vi "IFF_OneLine.vi"(0 "Ztest":dbl, 1 "Slices":cluster{"HighSlice":T1[], "LowSlice":T1[]}, 2 "TriangleInfo":T4, 5 "Sampling":T3, 7 "X":cluster{"Xmin":dbl, "Xmax":dbl}, 9 "DirVecs":dbl[][](array[numeric]), 11 "Y":dbl, 12 "PixSize(mm)":dbl) -> (4 "LineOut":dbl[](array[numeric]))   [LabVIEW 2014]
uses:
  TypeDefs/Poly2DwSlope.ctl
  TypeDefs/Point2DwSlope.ctl
  <vilib>/Analysis/baseanly.llb/Mean (DBL).vi
  <vilib>/Analysis/NI_AALBase.lvlib
panel:
  out "Waveform Graph":dbl[](graph)
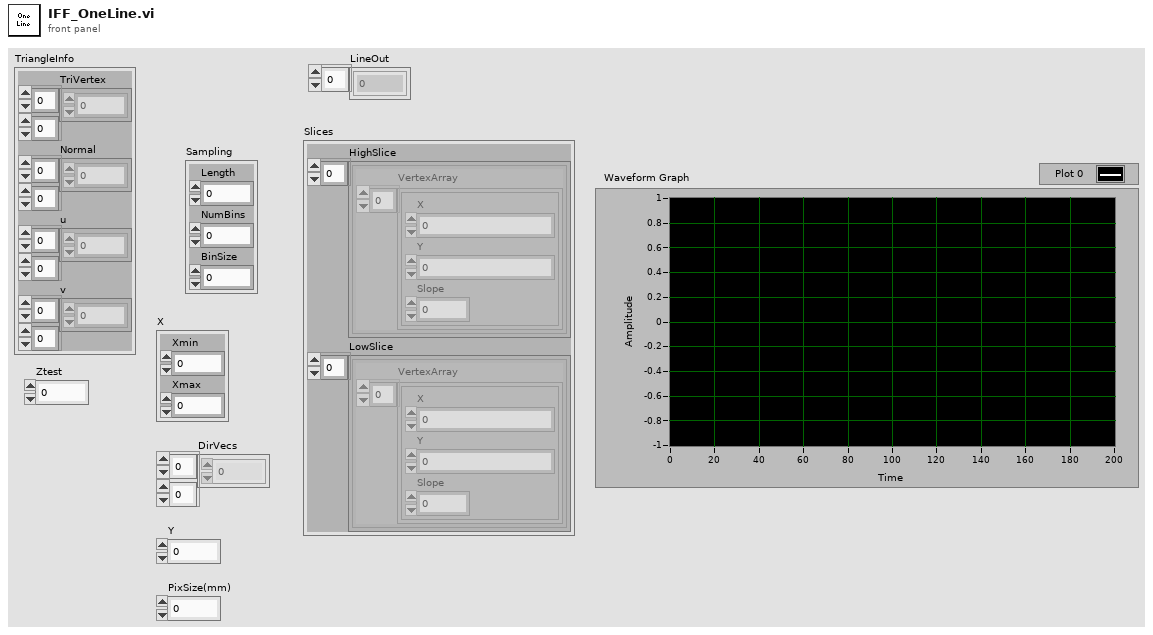
[diagram p1: front panel]
types:
  T1 = typedef "Poly2DwSlope.ctl" = cluster{"VertexArray":T2[]}
  T2 = typedef "Point2DwSlope.ctl" = cluster{"X":sgl, "Y":sgl, "Slope":dbl}
  T3 = cluster{"Length":dbl, "NumBins":dbl, "BinSize":dbl}
  T4 = cluster{"TriVertex":dbl[][], "Normal":dbl[][], "u":dbl[][], "v":dbl[][]}
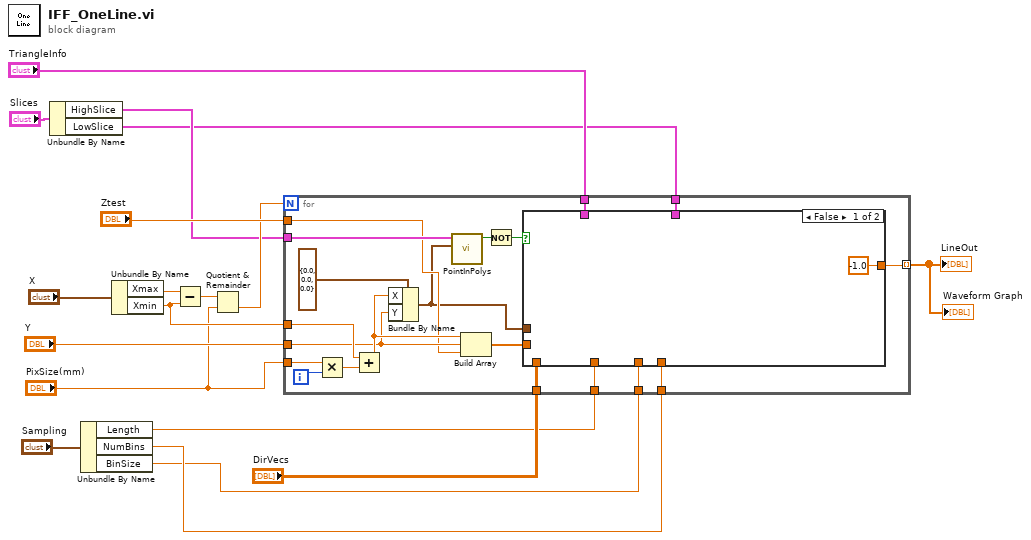
[diagram p0: block diagram]
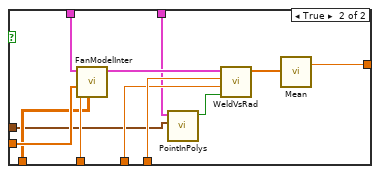
[diagram p2: hidden frame]
diagram:
  n1 = Unbundle By Name("Slices") -> ("HighSlice"=w3:T1[], "LowSlice"=w2:T1[])
  n2 = Unbundle By Name("Sampling") -> ("Length"=w7:dbl, "NumBins"=w6:dbl, "BinSize"=w5:dbl)
  n3 = Unbundle By Name("X") -> ("Xmax"=w17:dbl, "Xmin"=w18:dbl)
  n4 = Subtract(x=w17, y=w18) -> (x-y=w9:dbl)
  n5 = Quotient & Remainder(x=w9, y="PixSize(mm)") -> (floor(x/y)=w11:dbl)  [unwired: 1 out]
  n6 = for {
    N: w11 -> [_]
    tunnel: w3 -> [w38]
    tunnel: "PixSize(mm)" -> [w36]
    tunnel: w18 -> [w34]
    tunnel: "Y" -> [w27]
    tunnel: "Ztest" -> [w26]
    tunnel: w7 -> [w30]
    tunnel: "DirVecs" -> [w29]
    tunnel: w6 -> [w24]
    tunnel: w5 -> [w23]
    tunnel: w2 -> [w22]
    tunnel: [w20] -> w1 mode=indexing
    tunnel: "TriangleInfo" -> [w19]
    i -> [w37]
    n7 = Multiply(x=w36, y=w37) -> (x*y=w35:dbl)
    n8 = Add(x=w34, y=w35) -> (x+y=w28:dbl)
    n9 = Bundle By Name(cluster=T2 {"X"=0.0, "Y"=0.0, "Slope"=0.0} ("Point2D"), "X"=w28, "Y"=w27) -> (w21:T2)
    n10 = call "PointInPolys.vi"("Point2D"=w21, "Polys"=w38) -> ("Outside"=w32:bool)  [unwired: 9 in]
    n11 = Build Array(w28, w27, w26) -> (w25:dbl[])
    n12 = Not(x=w32) -> (.not. x?=w31:bool)
    n13 = case shown="False" w31 {
      tunnel: w25 -> [_ w51]
      tunnel: w30 -> [_ w50]
      tunnel: w29 -> [_ w49]
      tunnel: w24 -> [_ w47]
      tunnel: w23 -> [_ w46]
      tunnel: w22 -> [_ w45]
      tunnel: w21 -> [_ w44]
      tunnel: [-1.0 ("mean") w41] -> w20
      tunnel: w19 -> [_ w40]
      frame False {
      }
      frame True {
        n14 = call "FanModelInter.vi"("DirVecs"=w49, "Length"=w50, "Point"=w51, "TriangleInfo"=w40) -> ("Dists"=w48:cluster{dbl[]}[])  [unwired: 6 in, 1 out]
        n15 = call "PointInPolys.vi"("Point2D"=w44, "Polys"=w45) -> ("Outside"=w43:bool)  [unwired: 9 in]
        n16 = call "WeldVsRad.vi"("Outside"=w43, "BinSize (mm)"=w46, "NumBins"=w47, "Dists"=w48) -> ("WeldVsRadius"=w42:dbl[])  [unwired: 7 in]
        n17 = call-poly <vilib>:"Mean.vi"("X"=w42) -> ("mean"=w41:dbl)  [unwired: 1 out]
      }
    }
  }
  "LineOut" <- w1
  "Waveform Graph" <- w1
